vi "Driveless Path.vi"(1 "Path":path) -> (0 "Driveless Path":path)   [LabVIEW 2011]
doc: "Strips drive letter from path.\n\n\nVersion 1.0 - 03/09/2013\n\nPhaeron, Inc.\nwww.phaeron.com\ninfo@phaeron.com"
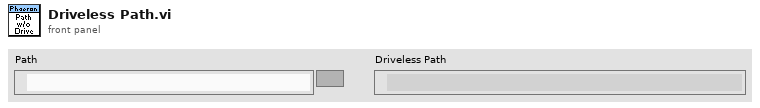
[diagram p1: front panel]
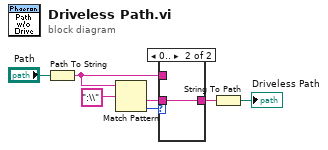
[diagram p0: block diagram]
diagram:
  n1 = Path To String(path="Path") -> (string=w7:string)
  n2 = Match Pattern(string=w7, regular expression=":\\") -> (after substring=w5:string, offset past match=w6:i32)  [unwired: 1 in, 2 out]
  n3 = case shown="0.." w6 {
    tunnel: w5 -> [_ w9]
    tunnel: w7 -> [w8 _]
    tunnel: [w8 w9] -> w2
    frame -1, Default {
    }
    frame 0.. {
    }
  }
  n4 = String To Path(string=w2) -> (path=→"Driveless Path":path)
